vi "CUST Disconnect PDC.vi"(11 "pseudoPdcId":i32) -> (3 "function return":i32)   [LabVIEW 2018, in "S3DK.lvlib" / "C37118-DLL.lvlib"]
doc: "STRONGRIDIEEEC37118DLL_API int __cdecl disconnectPdc( int32_t pseudoPdcId);"
uses:
  C37118-DLL.lvlib
  <vilib>/builds/S3DK Compiler/My Packed Library/StrongridDLL.dll
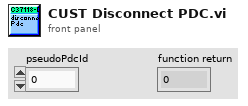
[diagram p1: front panel]
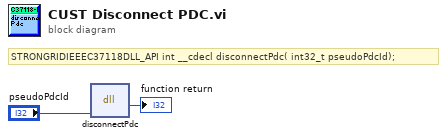
[diagram p0: block diagram]
diagram:
  # "STRONGRIDIEEEC37118DLL_API int __cdecl disconnectPdc( int32_t pseudoPdcId);"
  n1 = dll-call lib="C:/Program Files/National Instruments/LabVIEW 2018/vi.lib/builds/S3DK Compiler/My Packed Library/StrongridDLL.*" fn="disconnectPdc"("pseudoPdcId"="pseudoPdcId") -> (→"function return":i32)  [unwired: 4 in, 2 out]
